vi "Hello Print.vi"(8 "error in (no error)":errorcluster, 10 "Content":string, 11 "Demo Actor in":refnum<class "Demo Actor.lvclass">) -> (0 "error out":errorcluster, 3 "Demo Actor out":refnum<class "Demo Actor.lvclass">)   [LabVIEW 2020, in "First LV Actor.lvlib" / "Demo Actor.lvclass"]
uses:
  Demo Actor.lvclass
  C:/Program Files (x86)/National Instruments/LabVIEW 2020/vi.lib/ActorFramework/Actor/Actor.lvclass
  <vilib>/ActorFramework/Actor/Actor.lvclass/Actor.ctl
  <vilib>/ActorFramework/Message Enqueuer/Message Enqueuer.lvclass/Message Enqueuer.ctl
  <vilib>/ActorFramework/Message Enqueuer/Init from Existing Queue.vi
  <vilib>/ActorFramework/Message Enqueuer/Enqueue.vi
  <vilib>/ActorFramework/Stop Msg/Stop Msg.lvclass
  C:/Program Files (x86)/National Instruments/LabVIEW 2020/vi.lib/ActorFramework/Message/Message.lvclass
  <vilib>/ActorFramework/Message Priority Queue/Priority Enqueue.vi
  <vilib>/ActorFramework/Message Enqueuer/Message Enqueuer.lvclass
  <vilib>/ActorFramework/Actor/Actor.lvclass
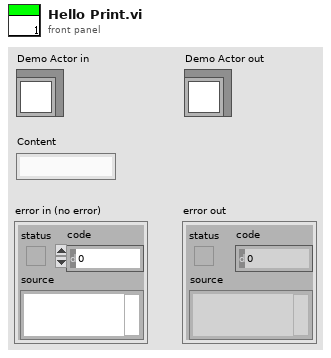
[diagram p1: front panel]
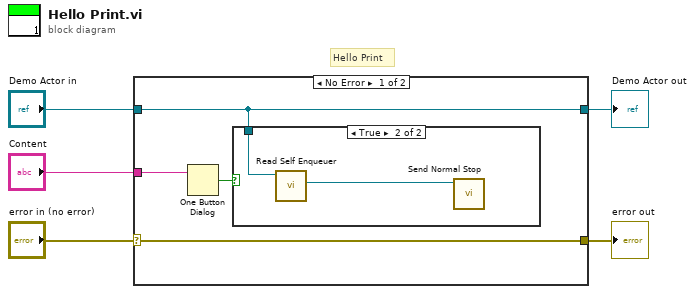
[diagram p0: block diagram]
diagram:
  # "Hello Print"
  n1 = case shown="No Error" "error in (no error)" {
    selector: "error in (no error)" -> [w9 w13]
    tunnel: [w9 w13] -> w4
    tunnel: [w7 w12] -> w2
    tunnel: "Demo Actor in" -> [w7 w12]
    tunnel: "Content" -> [w8 _]
    frame No Error {
      n2 = One Button Dialog(message=w8) -> (true=w6:bool)  [unwired: 1 in]
      n3 = case shown="True" w6 {
        tunnel: w7 -> [_ w11]
        frame False {
        }
        frame True {
          n4 = call <vilib>:"Read Self Enqueuer.vi"("Actor"=w11) -> ("Self Enqueuer"=w10:refnum<class "Message Enqueuer.lvclass">)  [unwired: 10 in]
          n5 = call <vilib>:"Send Normal Stop.vi"("Message Enqueuer"=w10) -> ()  [unwired: 10 in, 1 out]
        }
      }
    }
    frame Error {
    }
  }
  "error out" <- w4
  "Demo Actor out" <- w2
